vi "Input selector.vi"(6 "dt":dbl=0.0002807604, 8 "error in (no error)":errorcluster, 9 "Voltage INPUT2":dbl[](array[numeric]), 10 "Voltage INPUT1":dbl[](array[numeric]), 11 "Ring":u16(ring) items=["Both Inputs", "Input A", "Input B"]) -> (0 "error out":errorcluster, 1 "INPUT2 (Hz)":dbl=1234.889881600368 format="%0.3f", 2 "INPUT1 (Hz)":dbl=1234.889881600368 format="%0.3f", 3 "Sig Out":dynamicdata(graph), 4 "RAW":dynamicdata(graph), 5 "Product of CH1 an CH2":dbl[](array[numeric]))   [LabVIEW 2012]
uses:
  <vilib>/measure/matone.llb/Extract Single Tone Information 1 Chan.vi
  <vilib>/Analysis/2dsp.llb/Real FFT.vi
  <vilib>/measure/NI_MAPro.lvlib
  <vilib>/Analysis/NI_AALPro.lvlib
panel:
  out "Waveform Graph":dbl[](graph)
  in  "Export mode":u16(ring) items=["Fastest computation", "input signal—Input signal only", "detected signal—Single tone", "residual signal—Signal minus tone"]
  out "time":timestamp
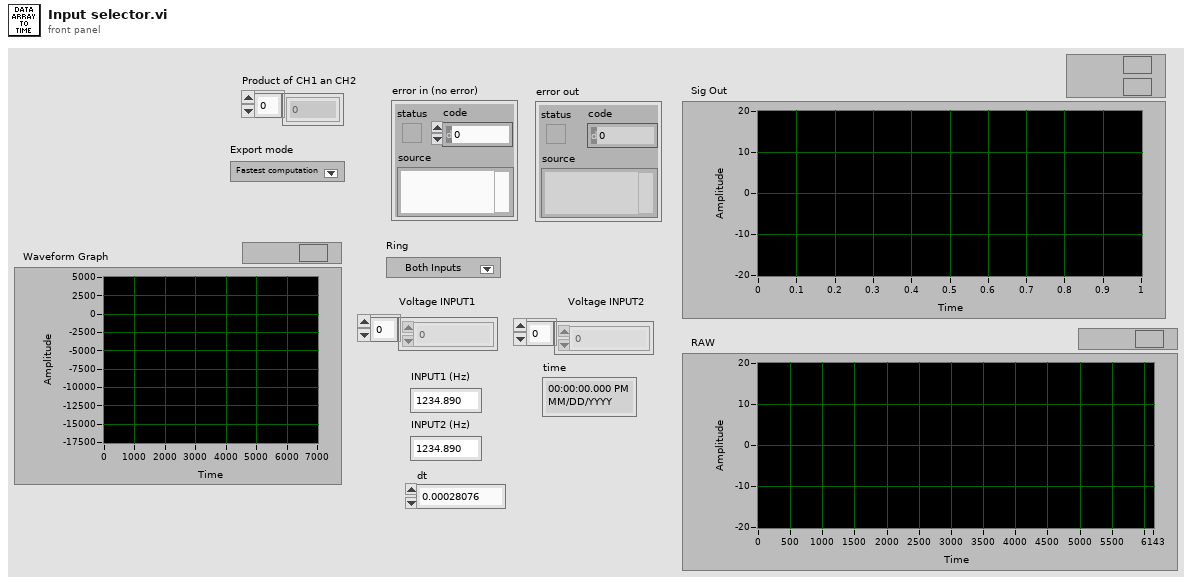
[diagram p1: front panel]
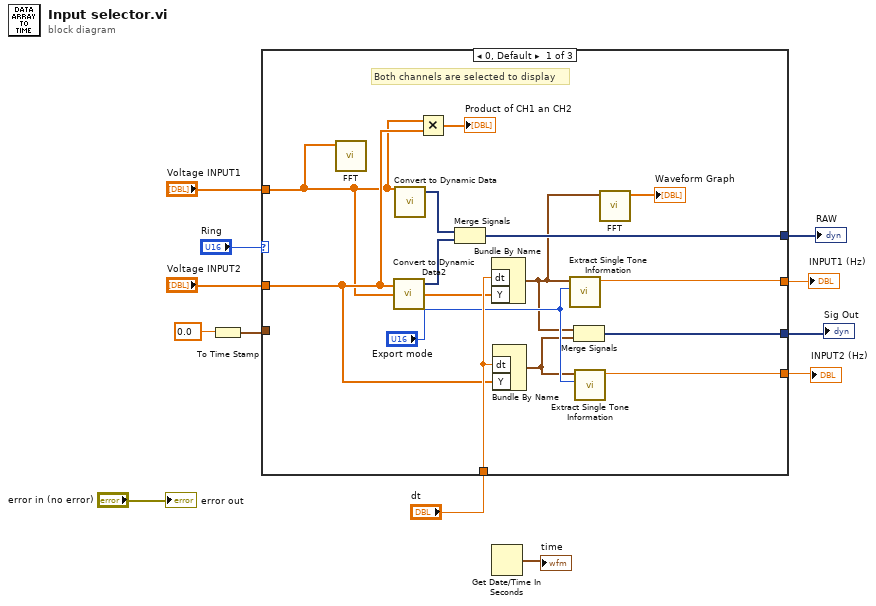
[diagram p0: block diagram]
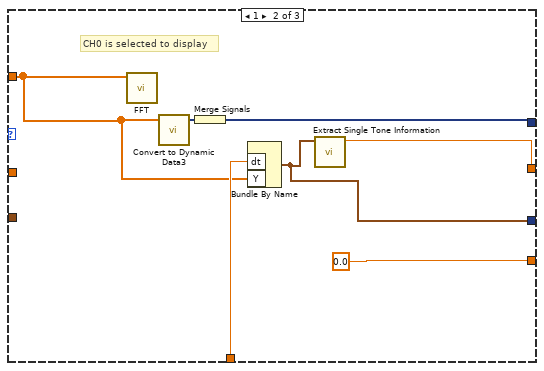
[diagram p2: hidden frame]
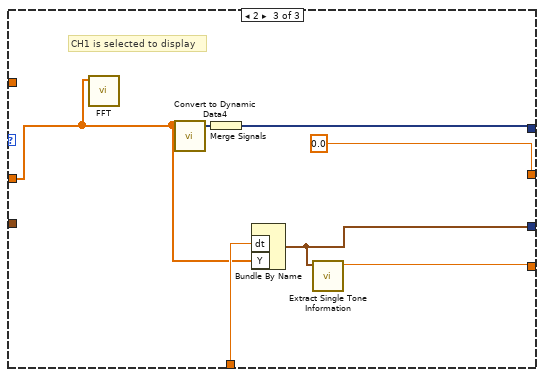
[diagram p3: hidden frame]
diagram:
  n1 = To Time Stamp(1:0.0 ("t0")) -> (0:w7:timestamp)
  n2 = case shown="0, Default" "Ring" {
    tunnel: "Voltage INPUT1" -> [w13 w27 _]
    tunnel: "Voltage INPUT2" -> [w19 _ w34]
    tunnel: [w24 w32 w40] -> w3
    tunnel: [w23 w28 w36] -> w8
    tunnel: "dt" -> [w22 w30 w38]
    tunnel: [w21 w29 0.0] -> w1
    tunnel: [w20 0.0 w35] -> w2
    tunnel: w7 -> [_ _ _]
    frame 0, Default {
      # "Both channels are selected to display"
      n3 = call-poly <vilib>:"FFT.vi"("X"=w13) -> ()  [unwired: 9 in, 2 out]
      n4 = call "Convert to Dynamic Data2"("Array"=w19) -> ("Dynamic Data Type"=w25:dynamicdata)  [unwired: 3 in]
      n5 = call "Convert to Dynamic Data"("Array"=w13) -> ("Dynamic Data Type"=w26:dynamicdata)  [unwired: 3 in]
      n6 = Multiply(x=w13, y=w19) -> (x*y=→"Product of CH1 an CH2":dbl[])
      n7 = Merge Signals(w26, w25) -> (w24:dynamicdata)
      n8 = Bundle By Name("dt"=w22, "Y"=w13) -> (w15:waveform(dbl))  [unwired: 1 in]
      n9 = Bundle By Name("dt"=w22, "Y"=w19) -> (w14:waveform(dbl))  [unwired: 1 in]
      n10 = call-poly <vilib>:"Extract Single Tone Information.vi"("export mode"="Export mode", "time signal in"=w15) -> ("detected frequency"=w21:dbl)  [unwired: 4 in, 5 out]
      n11 = Merge Signals(w15, w14) -> (w23:dynamicdata)
      n12 = call-poly <vilib>:"Extract Single Tone Information.vi"("export mode"="Export mode", "time signal in"=w14) -> ("detected frequency"=w20:dbl)  [unwired: 4 in, 5 out]
      n13 = call-poly <vilib>:"FFT.vi"("X"=w15) -> ("FFT {X}"=→"Waveform Graph":cdb[])  [unwired: 9 in, 1 out]
    }
    frame 1 {
      # "CH0 is selected to display"
      n14 = call-poly <vilib>:"FFT.vi"("X"=w27) -> ()  [unwired: 9 in, 2 out]
      n15 = call "Convert to Dynamic Data3"("Array"=w27) -> ("Dynamic Data Type"=w33:dynamicdata)  [unwired: 3 in]
      n16 = Merge Signals(w33) -> (w32:dynamicdata)
      n17 = Bundle By Name("dt"=w30, "Y"=w27) -> (w28:waveform(dbl))  [unwired: 1 in]
      n18 = call-poly <vilib>:"Extract Single Tone Information.vi"("time signal in"=w28) -> ("detected frequency"=w29:dbl)  [unwired: 5 in, 5 out]
    }
    frame 2 {
      # "CH1 is selected to display"
      n19 = call-poly <vilib>:"FFT.vi"("X"=w34) -> ()  [unwired: 9 in, 2 out]
      n20 = call "Convert to Dynamic Data4"("Array"=w34) -> ("Dynamic Data Type"=w39:dynamicdata)  [unwired: 3 in]
      n21 = Merge Signals(w39) -> (w40:dynamicdata)
      n22 = Bundle By Name("dt"=w38, "Y"=w34) -> (w36:waveform(dbl))  [unwired: 1 in]
      n23 = call-poly <vilib>:"Extract Single Tone Information.vi"("time signal in"=w36) -> ("detected frequency"=w35:dbl)  [unwired: 5 in, 5 out]
    }
  }
  "Sig Out" <- w8
  "RAW" <- w3
  "INPUT2 (Hz)" <- w2
  "INPUT1 (Hz)" <- w1
  n24 = Get Date/Time In Seconds() -> (seconds since 1Jan1904=→"time":timestamp)
  "error out" <- "error in (no error)"
